vi "UltraHarp Main.vi"() -> ()   [LabVIEW 2014]
uses:
  <vilib>/rvi/Emulation/niFpgaGetClockAttributes.vi
  <vilib>/rvi/Emulation/niFpgaSctlEmulationGetInTimedLoop.vi
  <vilib>/rvi/Emulation/niFpgaEmulationReportErrorSimple.vi
  <vilib>/rvi/eio/common/nirviEmuTemplateMethod_errors.vi
  <vilib>/rvi/Emulation/niFpgaCriticalErrorInLSC.vi
  <vilib>/rvi/Emulation/niFpgaProcessEmulError.vi
  <vilib>/eio/EIONode/EIONode.xnode
panel:
  out "Return Pulse Period 3":u32
  in  "Volume scaling":fxp<+/-,64,32>
  out "Return Pulse Period 4":u32
  out "Return Pulse Period 2":u32
  in  "Trigger pulse interval (mSec)":u32=200
  out "Return Pulse Period":u32
  in  "stop":bool
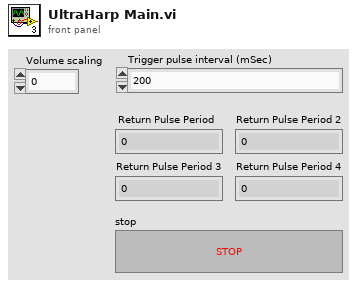
[diagram p1: front panel]
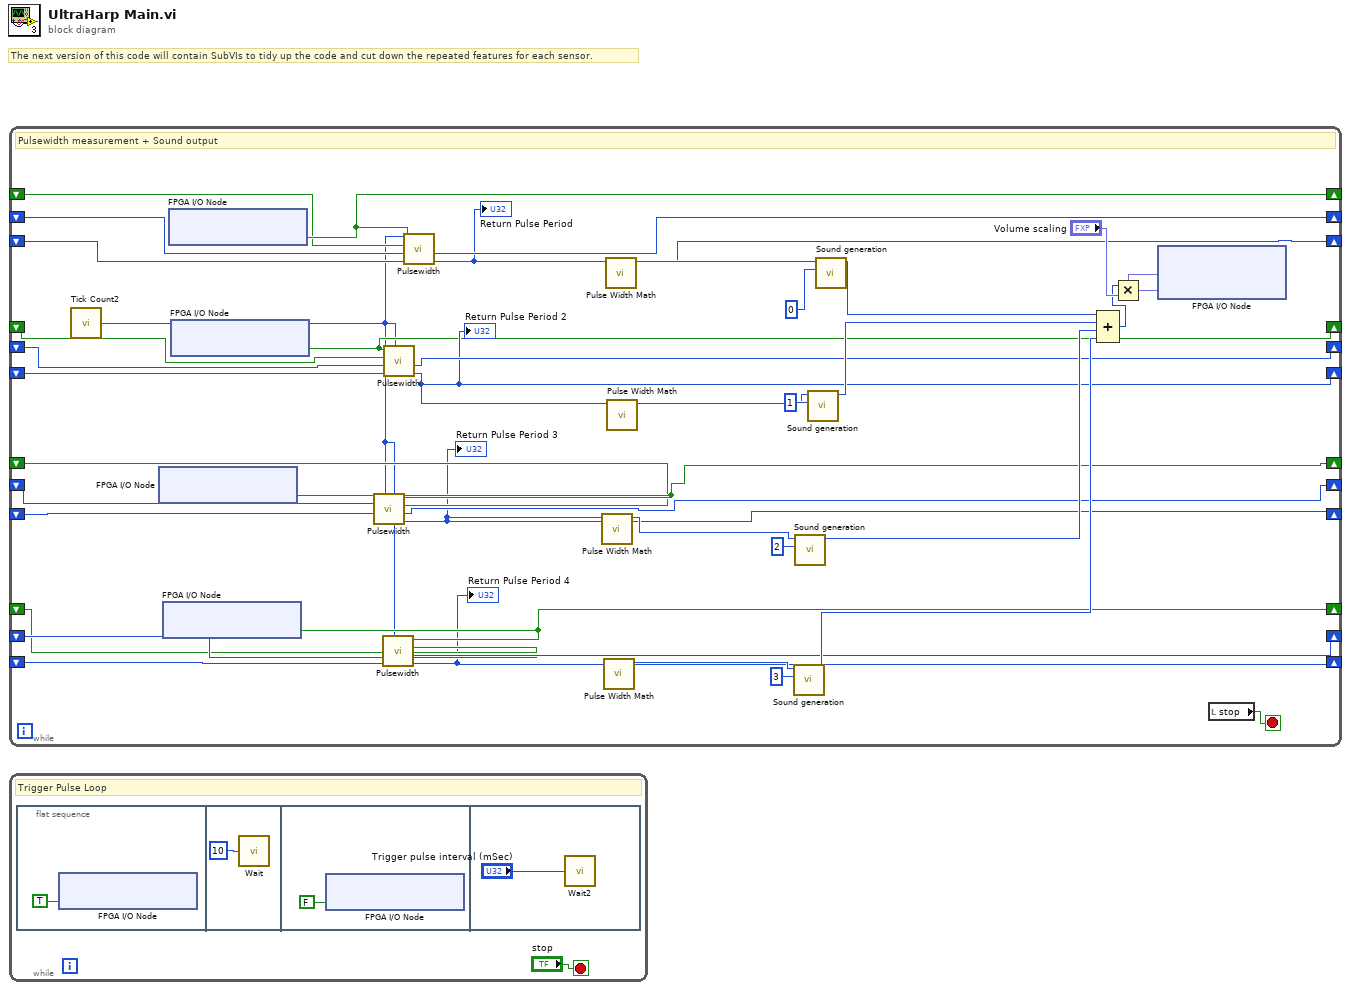
[diagram p0: block diagram]
diagram:
  # "The next version of this code will contain SubVIs to tidy up the code and cut down the repeated features for each sensor."
  n1 = while "Pulsewidth Measurement + Sound Output" {
    shift-left: _ -> [w4]
    shift-right: [w5] -> _
    shift-left: _ -> [w7]
    shift-right: [w6] -> _
    shift-left: _ -> [w8]
    shift-right: [w9] -> _
    shift-right: [w10] -> _
    shift-left: _ -> [w11]
    shift-right: [w15] -> _
    shift-left: _ -> [w12]
    shift-right: [w14] -> _
    shift-left: _ -> [w13]
    shift-right: [w19] -> _
    shift-left: _ -> [w16]
    shift-right: [w20] -> _
    shift-left: _ -> [w17]
    shift-right: [w3] -> _
    shift-left: _ -> [w18]
    shift-right: [w22] -> _
    shift-left: _ -> [w21]
    shift-right: [w24] -> _
    shift-left: _ -> [w23]
    shift-right: [w1] -> _
    shift-left: _ -> [w25]
    stop <- w41 stop-if-true
    # "Pulsewidth measurement + Sound output"
    n2 = call "Tick Count2"() -> ("Tick Count(uSec)"=w2:u32)
    n3 = xnode "FPGA I/O Node"() -> ("ConnectorC/DIO1"=w19:bool)  [unwired: 1 in, 1 out]
    n4 = xnode "FPGA I/O Node"() -> ("ConnectorC/DIO0"=w22:bool)  [unwired: 1 in, 1 out]
    n5 = xnode "FPGA I/O Node"() -> ("ConnectorC/DIO3"=w9:bool)  [unwired: 1 in, 1 out]
    n6 = xnode "FPGA I/O Node"() -> ("ConnectorC/DIO2"=w10:bool)  [unwired: 1 in, 1 out]
    n7 = call "Pulsewidth.vi"("Current Tick count"=w2, "Previous Updated Pulsewidth in"=w18, "Current Pulse Width In"=w17, "Prev. Echo Line State"=w16, "Echo Line State"=w19) -> ("Updated Pulsewidth out"=w3:u32, "Current Pulsewidth out"=w20:u32)  [unwired: 5 in]
    "Return Pulse Period 3" <- w3
    n8 = call "Pulsewidth.vi"("Current Tick count"=w2, "Previous Updated Pulsewidth in"=w25, "Current Pulse Width In"=w23, "Prev. Echo Line State"=w21, "Echo Line State"=w22) -> ("Updated Pulsewidth out"=w1:u32, "Current Pulsewidth out"=w24:u32)  [unwired: 5 in]
    "Return Pulse Period 4" <- w1
    n9 = call "Pulsewidth.vi"("Current Tick count"=w2, "Previous Updated Pulsewidth in"=w13, "Current Pulse Width In"=w12, "Prev. Echo Line State"=w11, "Echo Line State"=w10) -> ("Updated Pulsewidth out"=w14:u32, "Current Pulsewidth out"=w15:u32)  [unwired: 5 in]
    "Return Pulse Period 2" <- w14
    n10 = call "Pulsewidth.vi"("Current Tick count"=w2, "Previous Updated Pulsewidth in"=w4, "Current Pulse Width In"=w7, "Prev. Echo Line State"=w8, "Echo Line State"=w9) -> ("Updated Pulsewidth out"=w5:u32, "Current Pulsewidth out"=w6:u32)  [unwired: 5 in]
    "Return Pulse Period" <- w5
    n11 = call "Pulse Width Math.vi"("Pulse Width In"=w3) -> ("Numeric"=w27:i32)  [unwired: 10 in]
    n12 = call "Pulse Width Math.vi"("Pulse Width In"=w1) -> ("Numeric"=w26:i32)  [unwired: 10 in]
    n13 = call "Pulse Width Math.vi"("Pulse Width In"=w5) -> ("Numeric"=w29:i32)  [unwired: 10 in]
    n14 = call "Pulse Width Math.vi"("Pulse Width In"=w14) -> ("Numeric"=w28:i32)  [unwired: 10 in]
    n15 = call "Sound generation.vi"("sensor selector"=3, "cm distance"=w26) -> ("sine out"=w31:i16)  [unwired: 9 in]
    n16 = call "Sound generation.vi"("sensor selector"=2, "cm distance"=w27) -> ("sine out"=w33:i16)  [unwired: 9 in]
    n17 = call "Sound generation.vi"("sensor selector"=1, "cm distance"=w28) -> ("sine out"=w34:i16)  [unwired: 9 in]
    n18 = call "Sound generation.vi"("sensor selector"=0, "cm distance"=w29) -> ("sine out"=w35:i16)  [unwired: 9 in]
    n19 = Compound Arithmetic op=ADD(w35, w34, w33, w31) -> (w30:i16)
    n20 = Multiply(x=w30, y="Volume scaling") -> (x*y=w40:fxp<+/-,64,48>)
    n21 = xnode "FPGA I/O Node"("AudioOut/Left"=w40, "AudioOut/Right"=w40) -> ()  [unwired: 2 in, 2 out]
    n22 = local read "stop"() -> (w41:bool)
  }
  n23 = while {
    stop <- "stop" stop-if-true
    # "Trigger Pulse Loop"
    n24 = flat-sequence {
      frame #0 {
        n25 = xnode "FPGA I/O Node"("ConnectorC/DIO7"=TRUE ("ConnectorC/DIO6")) -> ()  [unwired: 1 in, 1 out]
      }
      frame #1 {
        n26 = call "Wait"("Count(uSec)"=u32 10) -> ()  [unwired: 1 out]
      }
      frame #2 {
        n27 = xnode "FPGA I/O Node"("ConnectorC/DIO7"=FALSE ("ConnectorC/DIO6")) -> ()  [unwired: 1 in, 1 out]
      }
      frame #3 {
        n28 = call "Wait2"("Count(mSec)"="Trigger pulse interval (mSec)") -> ()  [unwired: 1 out]
      }
    }
  }
